vi "Get Coordinates.vi"(8 "error in (no error)":errorcluster, 9 "Plot ID":i32, 11 "3D Scatter.lvclass in":refnum<class "3D Scatter.lvclass">) -> (0 "error out":errorcluster, 1 "Coordinates System":enum16{"Cartesian", "Cylindrical", "Spherical"}(ring), 3 "3D Scatter.lvclass out":refnum<class "3D Scatter.lvclass">)   [LabVIEW 2020, in "3D Scatter.lvclass"]
uses:
  <vilib>/Math Plots/3D Math Plots/3D Scatter/3D Scatter/3D Scatter.lvclass
  <vilib>/Math Plots/3D Math Plots/3D Scatter/3D Scatter/3D Scatter.lvclass/3D Scatter.ctl
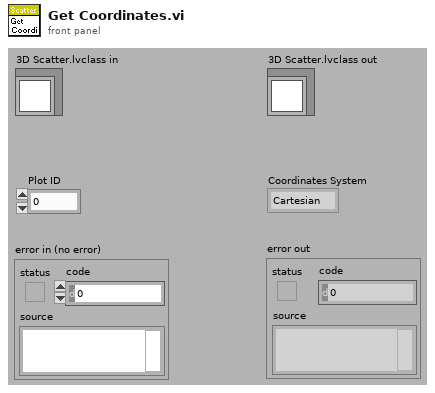
[diagram p1: front panel]
types:
  T1 = typedef "3D Scatter.lvclass/3D Scatter Property Array.ctl" = T2[]
  T2 = typedef "3D Scatter.lvclass/3D Scatter Property.ctl" = cluster{"General Property":cluster{"Plot Name":string, "Coordinate System":enum16{"Cartesian", "Cylindrical", "Spherical"}, "Opacity":sgl}, "Projection Property":cluster{"Draw XY":bool, "Draw YZ":bool, "Draw XZ":bool}, "Plot Property":cluster{"Sprite Type":T3, "Point Size":sgl, "Color Ramp Cluster":T4}}
  T3 = typedef "3D Plot.lvclass/Sprite Type.ctl" = enum16{"None", "Empty Square", "Solid Square", "Empty Diamond", "Solid Diamond", "Empty Circle", "Solid Circle", "Asterisk", "Bold X", "Wireframe Sphere", "Solid Sphere", "Wireframe Cube", "Solid Cube"}
  T4 = typedef "3D Plot.lvclass/Color Ramp Cluster.ctl" = cluster{"Color Ramp Style":enum16{"None", "Shaded", "Color spectrum", "Grey scale", "Custom"}, "Color Ramp Array":u32[], "Color Ramp Index":i32[], "Interpolate?":bool, "Logarithm?":bool}
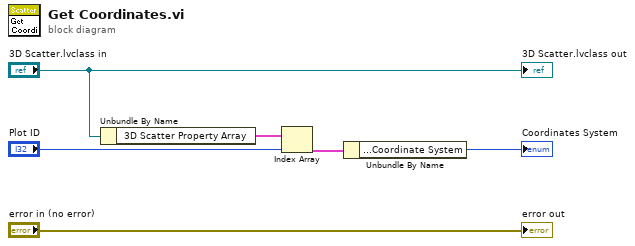
[diagram p0: block diagram]
diagram:
  n1 = Unbundle By Name("3D Scatter.lvclass in") -> ("3D Scatter Property Array"=w6:T1)
  n2 = Index Array(array=w6, index="Plot ID") -> (element=w5:T2)
  n3 = Unbundle By Name(w5) -> ("General Property.Coordinate System"=→"Coordinates System":enum16{"Cartesian", "Cylindrical", "Spherical"})
  "3D Scatter.lvclass out" <- "3D Scatter.lvclass in"
  "error out" <- "error in (no error)"
